vi "TRDU_max.vi"() -> ()   [LabVIEW 2020]
panel:
  in  "TRDU_max":dbl
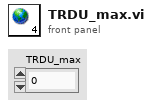
[diagram p1: front panel]
diagram:
